vi "Test Settings UI.vi"() -> ()   [LabVIEW 2020, in "Output Sequencer.lvlib" / "Settings UI.lvclass"]
uses:
  Settings UI.lvclass
  Settings UI.lvclass/Settings UI.ctl
  Output Sequencer/Types/UI Ref.ctl
  Output Sequencer/Output Sequencer.lvclass
  70c0feee-f92b-491b-951b-ba91555f4af3.vi
  Settings UI.vi
  Output Sequencer/Types/Event Type.ctl
  Output Sequencer/Types/UI Event.ctl
  Types/Step Settings.ctl
  Types/Settings.ctl
panel:
  in  "Digital Channels":string[](array[string])=["Dev1/port0/line0", "Start Trigger"]
  in  "Analog Channels":string[](array[string])=["MyChan", "Dev1/ai0", "Test Chan"]
  out "Init Settings out":T1={"Plug-in Version"="", "Step Values"=[], "Only Execute When Test Running"=TRUE, "Reset Sequence When Test Starts"=TRUE, "Number of Sequence Steps"=0, "Num of Analog Channels"=0, "Num of Digital Channels"=0, "Delay Before Starting Sequence"=0.0, "Default Analog Values"=[], "Default Digital Values"=[], "Max Iterations"=0, "Use last value when stopped"=FALSE, "Prioritize exact values"=FALSE, "Enable advanced step timing"=FALSE, "Enable step conditions"=FALSE, "Show confirmation dialogs"=FALSE, "Start condition"="", "Enable re-triggering"=FALSE, "Stop condition"=""}
  in  "Init Settings JSON":string="{\"Plug-in Version\":\"1.0\",\"Step Values\":[{\"Description\":\"Ramp up\",\"Precondition\":\"\",\"Duration\":1,\"Mode\":\"Wait for end of step\",\"Delay Between Values\":0,\"Analog Values\":[\"Last; Last + 5\"],\"Digital Values\":[],\"Postcondition\":\"\",\"On True\":\"\",\"On False\":\"\"},{\"Description\":\"Dwell\",\"Precondition\":\"\",\"Duration\":1,\"Mode\":\"Wait for end of step\",\"Delay Between Values\":0,\"Analog Values\":[\"Last\"],\"Digital Values\":[],\"Postcondition\":\"\",\"On True\":\"\",\"On False\":\"\"},{\"Description\":\"Ramp down\",\"Precondition\":\"\",\"Duration\":1,\"Mode\":\"Wait for end of step\",\"Delay Between Values\":0,\"Analog Values\":[\"Last; Last - 5\"],\"Digital Values\":[],\"Postcondition\":\"\",\"On True\":\"\",\"On False\":\"\"}],\"Only Execute When Test Running\":false,\"Reset Sequence When Test Starts\":true,\"Number of Sequence Steps\":3,\"Num of Analog Channels\":1,\"Num of Digital Channels\":0,\"Delay Before Starting Sequence\":0,\"Default Analog Values\":[0],\"Default Digital Values\":[],\"Max Iterations\":0,\"Use last value when stopped\":true,\"Prioritize exact values\":false,\"Enable advanced step timing\":false,\"Enable step conditions\":true,\"Show confirmation dialogs\":false,\"Start condition\":\"\"}"
  in  "Load from JSON?":bool=TRUE
  out "Applied Settings out":T1={"Plug-in Version"="", "Step Values"=[], "Only Execute When Test Running"=TRUE, "Reset Sequence When Test Starts"=TRUE, "Number of Sequence Steps"=0, "Num of Analog Channels"=0, "Num of Digital Channels"=0, "Delay Before Starting Sequence"=0.0, "Default Analog Values"=[], "Default Digital Values"=[], "Max Iterations"=0, "Use last value when stopped"=FALSE, "Prioritize exact values"=FALSE, "Enable advanced step timing"=FALSE, "Enable step conditions"=FALSE, "Show confirmation dialogs"=FALSE, "Start condition"="", "Enable re-triggering"=FALSE, "Stop condition"=""}
  in  "Show UI":bool
  in  "Stop":bool
  out "Applied Settings JSON out":string="{\"Plug-in Version\":\"1.0\",\"Step Values\":[{\"Description\":\"Ramp up\",\"Precondition\":\"\",\"Duration\":1,\"Mode\":\"Wait for end of step\",\"Delay Between Values\":0,\"Analog Values\":[\"Last; Last + 5\"],\"Digital Values\":[],\"Postcondition\":\"\",\"On True\":\"\",\"On False\":\"\"},{\"Description\":\"Dwell\",\"Precondition\":\"\",\"Duration\":1,\"Mode\":\"Wait for end of step\",\"Delay Between Values\":0,\"Analog Values\":[\"Last\"],\"Digital Values\":[],\"Postcondition\":\"\",\"On True\":\"\",\"On False\":\"\"},{\"Description\":\"Ramp down\",\"Precondition\":\"\",\"Duration\":1,\"Mode\":\"Wait for end of step\",\"Delay Between Values\":0,\"Analog Values\":[\"Last; Last - 5\"],\"Digital Values\":[],\"Postcondition\":\"\",\"On True\":\"\",\"On False\":\"\"}],\"Only Execute When Test Running\":true,\"Reset Sequence When Test Starts\":true,\"Number of Sequence Steps\":3,\"Num of Analog Channels\":1,\"Num of Digital Channels\":0,\"Delay Before Starting Sequence\":0,\"Default Analog Values\":[0],\"Default Digital Values\":[],\"Max Iterations\":0,\"Use last value when stopped\":true,\"Prioritize exact values\":false,\"Enable advanced step timing\":false,\"Enable step conditions\":true}"
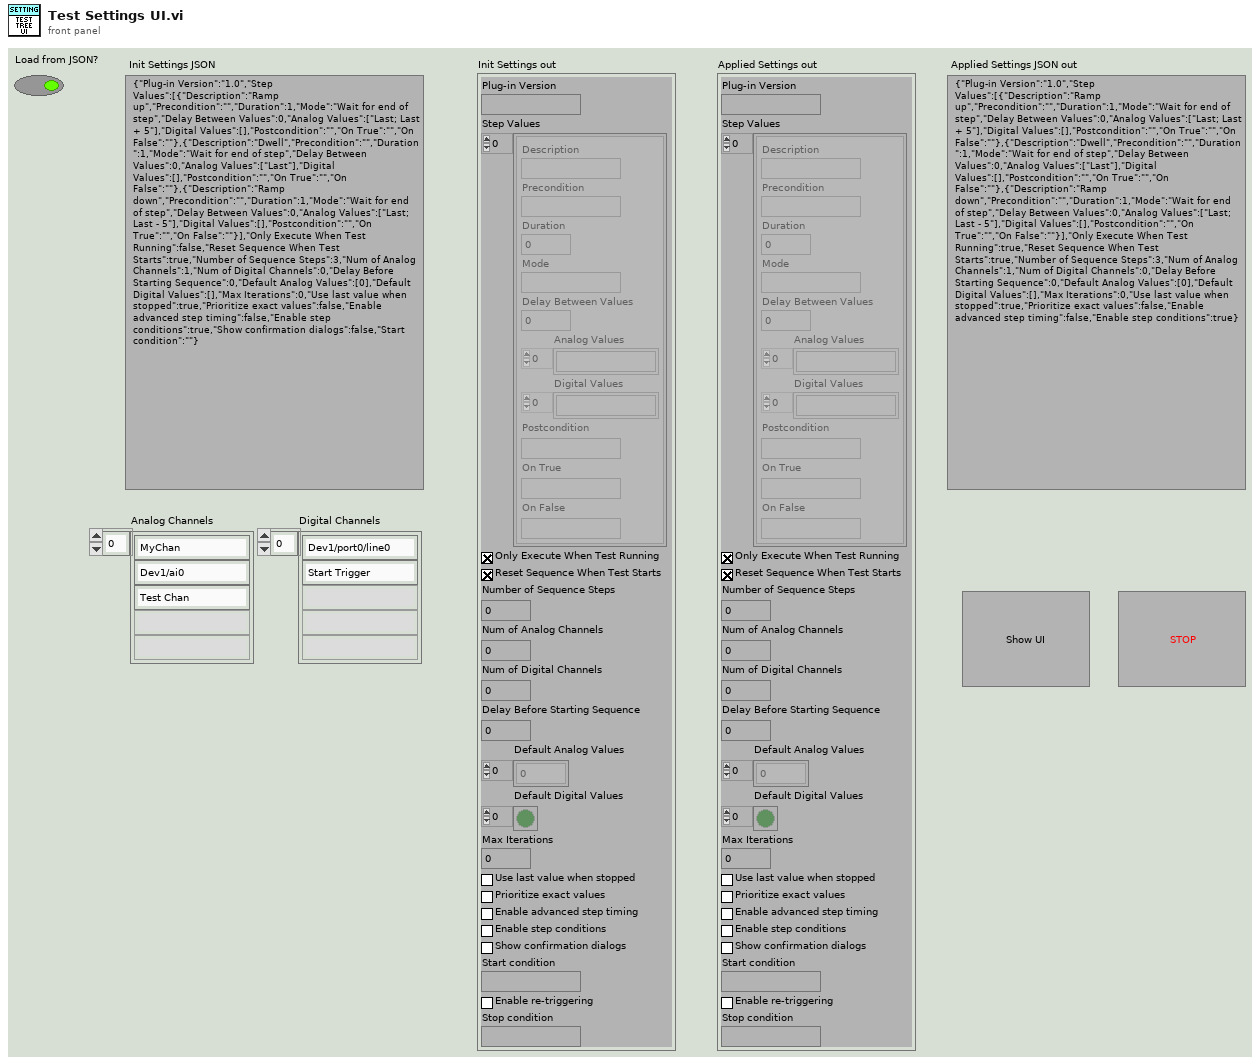
[diagram p1: front panel]
types:
  T1 = typedef "Output Sequencer.lvlib/Settings UI.lvclass/Settings.ctl" = cluster{"Plug-in Version":string, "Step Values":T2[], "Only Execute When Test Running":bool, "Reset Sequence When Test Starts":bool, "Number of Sequence Steps":i32, "Num of Analog Channels":i32, "Num of Digital Channels":i32, "Delay Before Starting Sequence":dbl, "Default Analog Values":dbl[], "Default Digital Values":bool[], "Max Iterations":u32, "Use last value when stopped":bool, "Prioritize exact values":bool, "Enable advanced step timing":bool, "Enable step conditions":bool, "Show confirmation dialogs":bool, "Start condition":string, "Enable re-triggering":bool, "Stop condition":string}
  T2 = typedef "Output Sequencer.lvlib/Settings UI.lvclass/Step Settings.ctl" = cluster{"Description":string, "Precondition":string, "Duration":dbl, "Mode":string, "Delay Between Values":dbl, "Analog Values":string[], "Digital Values":string[], "Postcondition":string, "On True":string, "On False":string}
  T3 = typedef "Output Sequencer.lvlib/Output Sequencer.lvclass/UI Ref.ctl" = refnum<vi>
  T4 = typedef "Output Sequencer.lvlib/Output Sequencer.lvclass/Event Type.ctl" = enum16{"Channel Update", "Test State Change", "Stop"}
  T5 = typedef "Output Sequencer.lvlib/Output Sequencer.lvclass/UI Event.ctl" = cluster{"Type":T4, "Data":variant}
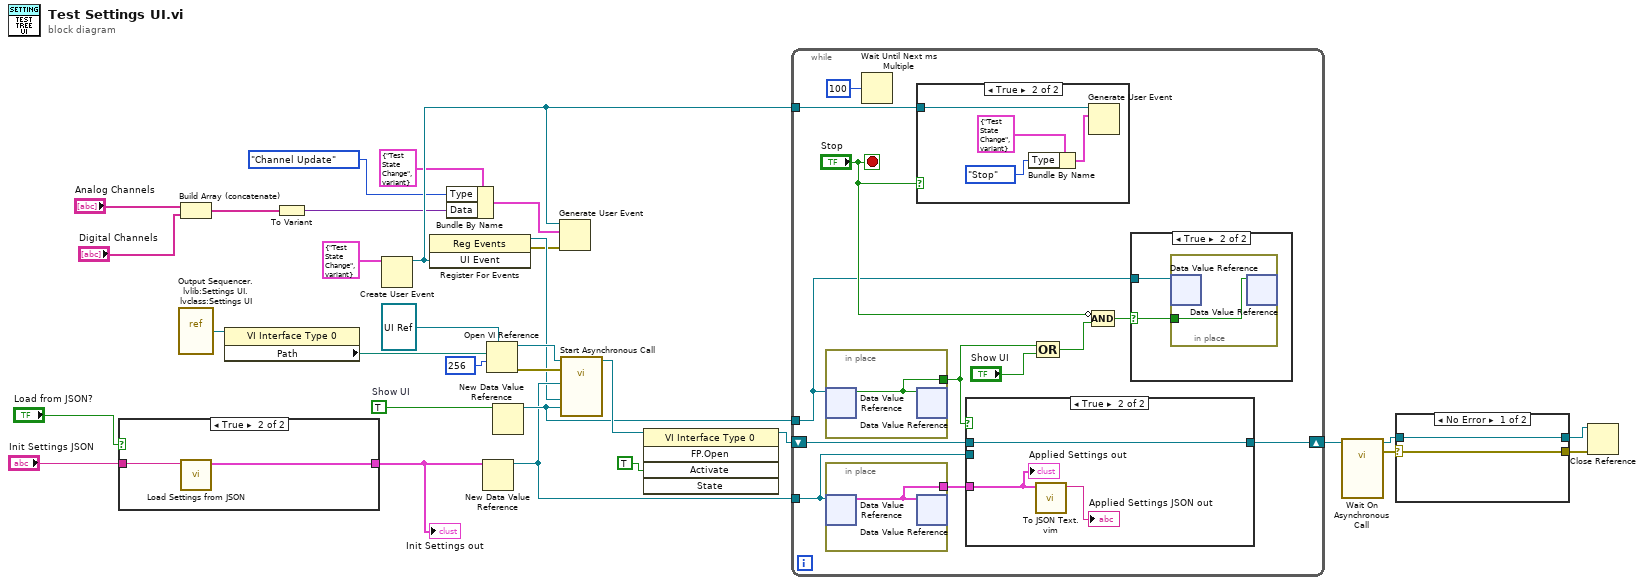
[diagram p0: block diagram]
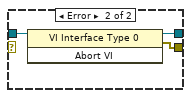
[diagram p2: hidden frame]
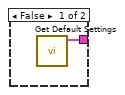
[diagram p3: hidden frame]
diagram:
  w19 = TRUE  # Show UI
  n1 = case shown="True" "Load from JSON?" {
    tunnel: [w32 w34] -> w17
    tunnel: "Init Settings JSON" -> [_ w33]
    frame False {
      n2 = call "Get Default Settings.vi"() -> ("Settings out"=w32:T1)  [unwired: 10 in, 1 out]
    }
    frame True {
      n3 = call "Load Settings from JSON.vi"("JSON String"=w33) -> ("Settings out"=w34:T1)  [unwired: 9 in, 1 out]
    }
  }
  "Init Settings out" <- w17
  n4 = vi-ref "Output Sequencer.lvlib:Settings UI.lvclass:Settings UI.vi"() -> (w20:refnum<vi>)
  n5 = Build Array (concatenate)("Analog Channels", "Digital Channels") -> (w12:string[])
  n6 = property class="VI Interface Type 0"(reference=w20) -> ("Path"=w30:path)  [unwired: 1 in, 2 out]
  n7 = To Variant(anything=w12) -> (Variant=w4:variant)
  n8 = Create User Event(user event datatype=T5 {"Type"=enum."Test State Change", "Data"=variant} ("UI Event")) -> (user event=w10:refnum<user-event>)  [unwired: 1 in, 1 out]
  n9 = register-events(w10) -> (reference out=w9:refnum<event-registration>, error out=w8:errorcluster)  [unwired: 2 in]
  n10 = Bundle By Name(cluster=T5 {"Type"=enum."Test State Change", "Data"=variant} ("UI Event"), "Type"=Event_Type."Channel Update", "Data"=w4) -> (w6:T5)
  n11 = New Data Value Reference(data value=w17) -> (data value reference=w16:refnum<data-value>)  [unwired: 1 in, 1 out]
  n12 = Open VI Reference(type specifier VI Refnum (for type only)=T3 refnum ("Cust UI"), vi path=w30, options=256) -> (vi reference=w21:T3, error out=w31:errorcluster)  [unwired: 3 in]
  n13 = New Data Value Reference(data value=w19) -> (data value reference=w18:refnum<data-value>)  [unwired: 1 in, 1 out]
  n14 = Generate User Event(user event=w10, event data cluster=w6, error in=w8) -> ()  [unwired: 1 in, 2 out]
  n15 = call-by-ref "Start Asynchronous Call"(reference=w21, error in=w31, "Show UI"=w18, "UI Event Registration"=w9, "Applied Settings"=w16) -> (reference out=w22:T3)  [unwired: 9 in, 1 out]
  n16 = invoke class="VI Interface Type 0" method="FP.Open"(reference=w22, "Activate"=TRUE ("Activate?")) -> (reference out=w11:T3)  [unwired: 3 in, 4 out]
  n17 = while {
    shift-right: [w44] -> w27
    shift-left: w11 -> [w45]
    tunnel: w16 -> [w40]
    tunnel: w10 -> [w43]
    tunnel: w18 -> [w35]
    stop <- "Stop" stop-if-true
    n18 = in-place {
      in-place-border: [w47] -> w36
      n19 = in-place-dvr #1(w35) -> (w47:bool)  [unwired: 1 out]
      n20 = in-place-dvr #1(w47) -> ()  [unwired: 2 out]
    }
    n21 = in-place {
      in-place-border: [w48] -> w42
      n22 = in-place-dvr #2(w40) -> (w48:T1)  [unwired: 1 out]
      n23 = in-place-dvr #2(w48) -> ()  [unwired: 2 out]
    }
    n24 = Wait Until Next ms Multiple(millisecond multiple=u32 100) -> ()  [unwired: 1 out]
    n25 = case shown="True" "Stop" {
      tunnel: w43 -> [_ w52]
      frame False {
      }
      frame True {
        n26 = Bundle By Name(cluster=T5 {"Type"=enum."Test State Change", "Data"=variant} ("UI Event"), "Type"=Event_Type."Stop") -> (w50:T5)
        n27 = Generate User Event(user event=w52, event data cluster=w50) -> ()  [unwired: 2 in, 2 out]
      }
    }
    n28 = case shown="True" w36 {
      tunnel: w45 -> [w56 w58]
      tunnel: [w56 w58] -> w44
      tunnel: w40 -> [_ _]
      tunnel: w42 -> [_ w57]
      frame False {
      }
      frame True {
        n29 = call "To JSON Text.vim"("Anything"=w57) -> ("<JSON>"=→"Applied Settings JSON out":string)  [unwired: 9 in, 1 out]
        "Applied Settings out" <- w57
      }
    }
    n30 = Compound Arithmetic op=OR(w36, "Show UI") -> (w39:bool)
    n31 = Compound Arithmetic op=AND(invert "Stop", w39) -> (w37:bool)
    n32 = case shown="True" w37 {
      selector: w37 -> [_ w54]
      tunnel: w35 -> [_ w53]
      frame False {
      }
      frame True {
        n33 = in-place {
          in-place-border: w54 -> [w55]
          n34 = in-place-dvr #3(w53) -> ()  [unwired: 2 out]
          n35 = in-place-dvr #3(w55) -> ()  [unwired: 2 out]
        }
      }
    }
  }
  n36 = call-by-ref "Wait On Asynchronous Call"(reference=w27) -> (reference out=w2:T3, error out=w3:errorcluster)  [unwired: 13 in]
  n37 = case shown="No Error" w3 {
    selector: w3 -> [w60 _]
    tunnel: w2 -> [w61 w64]
    tunnel: [w61 w63] -> w26
    tunnel: [w60 w62] -> w23
    frame No Error {
    }
    frame Error {
      n38 = invoke class="VI Interface Type 0" method="Abort VI"(reference=w64) -> (reference out=w63:T3, error out=w62:errorcluster)  [unwired: 2 in, 1 out]
    }
  }
  n39 = Close Reference(reference=w26, error in (no error)=w23) -> ()  [unwired: 1 out]
